vi "Terminal_PressureSystem_Display.vi"   [LabVIEW 2014]
types:
  T1 = cluster{"径向油缸加载压力":u16, "轴向油缸加载压力":u16, "油箱1油液温度":u16, "润滑油温度":u16, "油箱2油液温度":u16, "试验轴承供油压力":u16, "试验轴承供油流量":u16, "陪试轴承供油流量":u16, "陪试轴承供油压力":u16, "陪试轴承供油温度":u16, "液压子系统状态字":cluster{"加载单元":cluster{"供油过滤器堵塞报警":bool, "回油过滤器堵塞报警":bool, "液位过高报警":bool, "液位过低报警":bool}, "试验轴承单元":cluster{"加热装置异常报警":bool, "油箱1液位过高报警":bool, "油箱1液位过低报警":bool, "油箱2液位过高报警":bool, "油箱2液位过低报警":bool, "供油过滤器堵塞报警":bool, "循环回路过滤器堵塞报警":bool, "回油过滤器堵塞报警":bool}, "陪试轴承单元":cluster{"供油过滤器1堵塞报警":bool, "供油过滤器2堵塞报警":bool, "回油过滤器堵塞报警":bool, "油箱液位过高报警":bool, "油箱液位过低报警":bool}}}
  T2 = cluster{"径向油缸加载压力":u16, "轴向油缸加载压力":u16, "油箱1油液温度":u16, "润滑油温度":u16, "油箱2油液温度":u16, "试验轴承供油压力":u16, "试验轴承供油流量":u16, "陪试轴承供油流量":u16, "陪试轴承供油压力":u16, "陪试轴承供油温度":u16}
  T3 = cluster{"油箱1油液温度":dbl, "油箱2油液温度":dbl, "供油压力最小值":dbl, "供油压力最大值":dbl, "润滑油温度T2最小值":dbl, "润滑油温度T2最大值":dbl, "供油流量L1最小值":dbl, "供油流量L1最大值":dbl}
  T4 = cluster{"供油过滤器1堵塞报警":bool, "供油过滤器2堵塞报警":bool, "回油过滤器堵塞报警":bool, "油箱液位过高报警":bool, "油箱液位过低报警":bool}
  T5 = cluster{"供油过滤器堵塞报警":bool, "回油过滤器堵塞报警":bool, "液位过高报警":bool, "液位过低报警":bool}
  T6 = cluster{"加热装置异常报警":bool, "油箱1液位过高报警":bool, "油箱1液位过低报警":bool, "油箱2液位过高报警":bool, "油箱2液位过低报警":bool, "供油过滤器堵塞报警":bool, "循环回路过滤器堵塞报警":bool, "回油过滤器堵塞报警":bool}
  T7 = cluster{"润滑油温度T2最小值":dbl, "润滑油温度T2最大值":dbl, "润滑油温度":u16}
  T8 = cluster{"供油压力最小值":dbl, "供油压力最大值":dbl, "试验轴承供油压力":u16}
  T9 = cluster{"供油流量L1最小值":dbl, "供油流量L1最大值":dbl, "试验轴承供油流量":u16}
  T10 = cluster{cluster{"油箱1油液温度":dbl, "油箱1油液温度":u16}, cluster{"润滑油温度T2最小值":dbl, "润滑油温度T2最大值":dbl, "润滑油温度":u16}, cluster{"油箱2油液温度":dbl, "油箱2油液温度":u16}, cluster{"供油压力最小值":dbl, "供油压力最大值":dbl, "试验轴承供油压力":u16}, cluster{"供油流量L1最小值":dbl, "供油流量L1最大值":dbl, "试验轴承供油流量":u16}, "试验轴承单元":cluster{"加热装置异常报警":bool, "油箱1液位过高报警":bool, "油箱1液位过低报警":bool, "油箱2液位过高报警":bool, "油箱2液位过低报警":bool, "供油过滤器堵塞报警":bool, "循环回路过滤器堵塞报警":bool, "回油过滤器堵塞报警":bool}}
  T11 = cluster{"陪试轴承供油流量":u16, "陪试轴承供油压力":u16, "陪试轴承供油温度":u16, "陪试轴承单元":cluster{"供油过滤器1堵塞报警":bool, "供油过滤器2堵塞报警":bool, "回油过滤器堵塞报警":bool, "油箱液位过高报警":bool, "油箱液位过低报警":bool}}
  T12 = cluster{"径向油缸加载压力":u16, "轴向油缸加载压力":u16, "加载单元":cluster{"供油过滤器堵塞报警":bool, "回油过滤器堵塞报警":bool, "液位过高报警":bool, "液位过低报警":bool}}
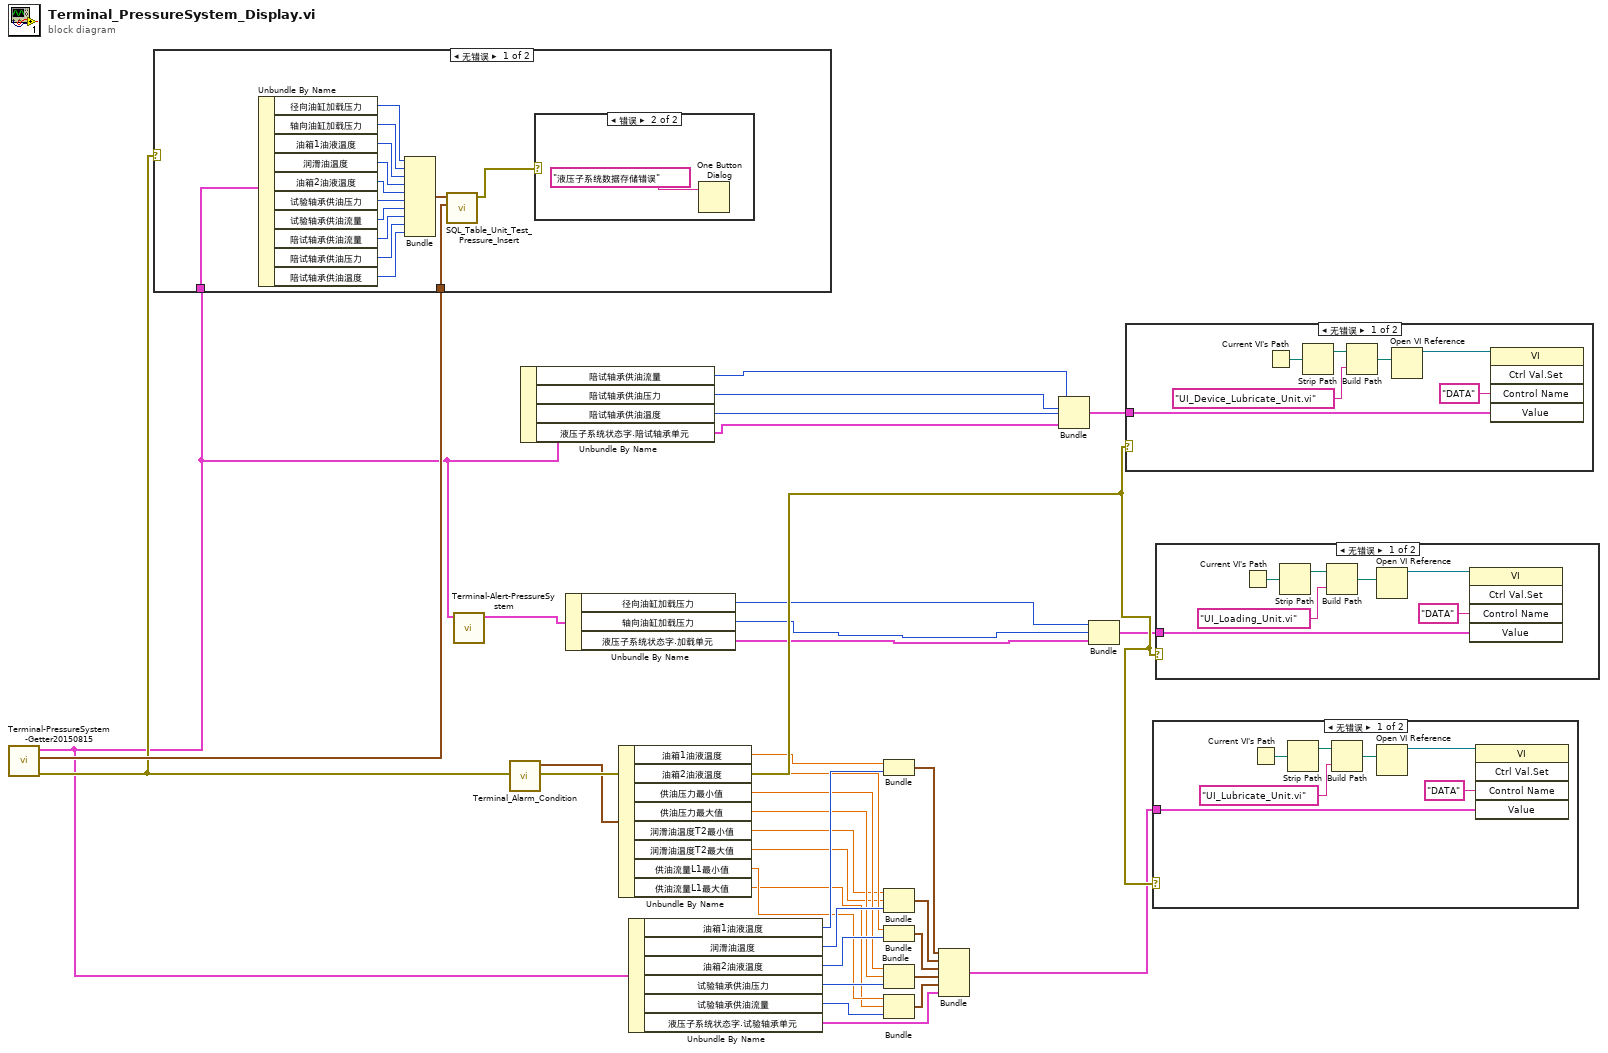
[diagram p0: block diagram]
diagram:
  n1 = call "Terminal-PressureSystem-Getter20150815.vi"() -> ("error out"=w32:errorcluster, "时间标识"=w33:timestamp, "设备信息"=w31:T1)  [unwired: 9 in]
  n2 = case shown="无错误" w32 {
    tunnel: w33 -> [w37 _]
    tunnel: w31 -> [w35 _]
    frame No Error {
      n3 = Unbundle By Name(w35) -> ("径向油缸加载压力"=w48:u16, "轴向油缸加载压力"=w47:u16, "油箱1油液温度"=w46:u16, "润滑油温度"=w45:u16, "油箱2油液温度"=w44:u16, "试验轴承供油压力"=w43:u16, "试验轴承供油流量"=w42:u16, "陪试轴承供油流量"=w41:u16, "陪试轴承供油压力"=w40:u16, "陪试轴承供油温度"=w39:u16)
      n4 = Bundle("径向油缸加载压力"=w48, "轴向油缸加载压力"=w47, "油箱1油液温度"=w46, "润滑油温度"=w45, "油箱2油液温度"=w44, "试验轴承供油压力"=w43, "试验轴承供油流量"=w42, "陪试轴承供油流量"=w41, "陪试轴承供油压力"=w40, "陪试轴承供油温度"=w39) -> (w38:T2)  [unwired: 1 in]
      n5 = call "SQL_Table_Unit_Test_Pressure_Insert.vi"("时间标识"=w37, "液压子系统数据"=w38) -> ("error out"=w36:errorcluster)  [unwired: 9 in]
      n6 = case shown="错误" w36 {
        frame No Error {
        }
        frame Error {
          n7 = One Button Dialog(message="液压子系统数据存储错误" ("消息")) -> ()  [unwired: 1 in, 1 out]
        }
      }
    }
    frame Error {
    }
  }
  n8 = call "Terminal-Alert-PressureSystem.vi"("液压子系统设备信息"=w31) -> ("液压子系统设备信息输出"=w34:T1)  [unwired: 10 in]
  n9 = call "Terminal_Alarm_Condition.vi"() -> ("试验轴承单元"=w14:T3)  [unwired: 11 in]
  n10 = Unbundle By Name(w31) -> ("陪试轴承供油流量"=w9:u16, "陪试轴承供油压力"=w8:u16, "陪试轴承供油温度"=w7:u16, "液压子系统状态字.陪试轴承单元"=w30:T4)
  n11 = Unbundle By Name(w34) -> ("径向油缸加载压力"=w5:u16, "轴向油缸加载压力"=w6:u16, "液压子系统状态字.加载单元"=w28:T5)
  n12 = Unbundle By Name(w14) -> ("油箱1油液温度"=w13:dbl, "油箱2油液温度"=w12:dbl, "供油压力最小值"=w11:dbl, "供油压力最大值"=w10:dbl, "润滑油温度T2最小值"=w4:dbl, "润滑油温度T2最大值"=w3:dbl, "供油流量L1最小值"=w2:dbl, "供油流量L1最大值"=w1:dbl)
  n13 = Unbundle By Name(w31) -> ("油箱1油液温度"=w26:u16, "润滑油温度"=w25:u16, "油箱2油液温度"=w24:u16, "试验轴承供油压力"=w23:u16, "试验轴承供油流量"=w22:u16, "液压子系统状态字.试验轴承单元"=w17:T6)
  n14 = Bundle("油箱1油液温度"=w13, "油箱1油液温度"=w26) -> (w15:cluster{"油箱1油液温度":dbl, "油箱1油液温度":u16})  [unwired: 1 in]
  n15 = Bundle("润滑油温度T2最小值"=w4, "润滑油温度T2最大值"=w3, "润滑油温度"=w25) -> (w21:T7)  [unwired: 1 in]
  n16 = Bundle("油箱2油液温度"=w12, "油箱2油液温度"=w24) -> (w20:cluster{"油箱2油液温度":dbl, "油箱2油液温度":u16})  [unwired: 1 in]
  n17 = Bundle("供油压力最小值"=w11, "供油压力最大值"=w10, "试验轴承供油压力"=w23) -> (w19:T8)  [unwired: 1 in]
  n18 = Bundle("供油流量L1最小值"=w2, "供油流量L1最大值"=w1, "试验轴承供油流量"=w22) -> (w18:T9)  [unwired: 1 in]
  n19 = Bundle(w15, w21, w20, w19, w18, "试验轴承单元"=w17) -> (w16:T10)  [unwired: 1 in]
  n20 = Bundle("陪试轴承供油流量"=w9, "陪试轴承供油压力"=w8, "陪试轴承供油温度"=w7, "陪试轴承单元"=w30) -> (w29:T11)  [unwired: 1 in]
  n21 = Bundle("径向油缸加载压力"=w5, "轴向油缸加载压力"=w6, "加载单元"=w28) -> (w27:T12)  [unwired: 1 in]
  n22 = case shown="无错误" w32 {
    tunnel: w29 -> [w50 _]
    frame No Error {
      n23 = Current VI's Path() -> (path=w54:path)
      n24 = Strip Path(path=w54) -> (stripped path=w55:path)  [unwired: 1 out]
      n25 = Build Path(base path=w55, name or relative path="UI_Device_Lubricate_Unit.vi") -> (appended path=w52:path)
      n26 = Open VI Reference(vi path=w52) -> (vi reference=w51:refnum<vi>)  [unwired: 5 in, 1 out]
      n27 = invoke class="VI" method="Ctrl Val.Set"(reference=w51, "Control Name"="DATA", "Value"=w50) -> ()  [unwired: 2 in, 5 out]
    }
    frame Error {
    }
  }
  n28 = case shown="无错误" w32 {
    tunnel: w16 -> [w57 _]
    frame No Error {
      n29 = Current VI's Path() -> (path=w61:path)
      n30 = Strip Path(path=w61) -> (stripped path=w62:path)  [unwired: 1 out]
      n31 = Build Path(base path=w62, name or relative path="UI_Lubricate_Unit.vi") -> (appended path=w59:path)
      n32 = Open VI Reference(vi path=w59) -> (vi reference=w58:refnum<vi>)  [unwired: 5 in, 1 out]
      n33 = invoke class="VI" method="Ctrl Val.Set"(reference=w58, "Control Name"="DATA", "Value"=w57) -> ()  [unwired: 2 in, 5 out]
    }
    frame Error {
    }
  }
  n34 = case shown="无错误" w32 {
    tunnel: w27 -> [w64 _]
    frame No Error {
      n35 = Current VI's Path() -> (path=w68:path)
      n36 = Strip Path(path=w68) -> (stripped path=w69:path)  [unwired: 1 out]
      n37 = Build Path(base path=w69, name or relative path="UI_Loading_Unit.vi") -> (appended path=w66:path)
      n38 = Open VI Reference(vi path=w66) -> (vi reference=w65:refnum<vi>)  [unwired: 5 in, 1 out]
      n39 = invoke class="VI" method="Ctrl Val.Set"(reference=w65, "Control Name"="DATA", "Value"=w64) -> ()  [unwired: 2 in, 5 out]
    }
    frame Error {
    }
  }
